vi "ex_setTdmProperty_I32.vi"(4 "Strings":string[](array[string]), 5 "Values":i32[](array[numeric]), 6 "Value":i32, 7 "Name":string) -> (3 "output cluster":T1)   [LabVIEW 2017]
uses:
  <vilib>/express/express shared/ExFile.llb/ex_TdmProperty.ctl
  <vilib>/express/express shared/ex_EditUserDefinedProperties/usiDataType.ctl
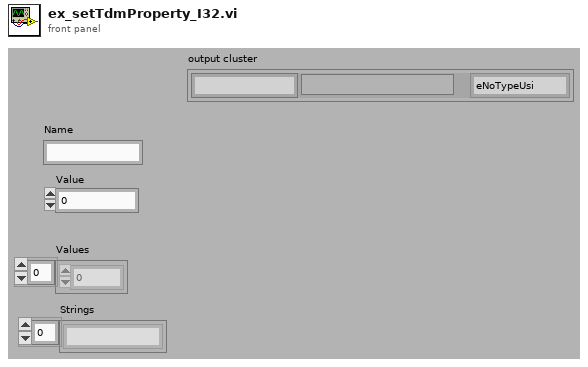
[diagram p1: front panel]
types:
  T1 = typedef "ex_TdmProperty.ctl" = cluster{"Name":string, "Type":T2, "Value":variant}
  T2 = typedef "usiDataType.ctl" = enum16{"eNoTypeUsi", "eInt8Usi", "eInt16Usi", "eInt32Usi", "eInt64Usi", "eUInt8Usi", "eUInt16Usi", "eUInt32Usi", "eUInt64Usi", "eFloat32Usi", "eFloat64Usi", "- 0", "- 1", "- 2", "- 3", "- 4", "- 5", "- 6", "- 7", "- 8", "- 9", "eString8Usi", "eString16Usi", "eStringUsi", "eEnumUsi", "- 10", "- 11", "- 12", "- 13", "- 14", "eTimeUsi", "- 15", "- 16", "- 17", "- 18", "- 19", "- 20", "- 21", "- 22", "- 23", "eInstanceUsi", "eStoreUsi"}
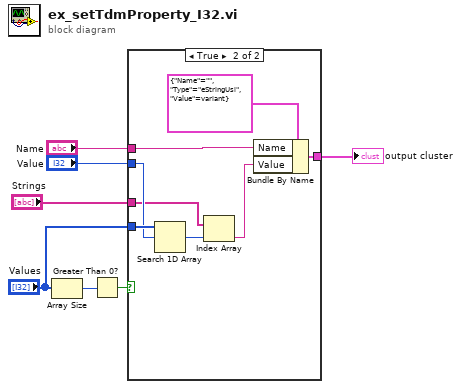
[diagram p0: block diagram]
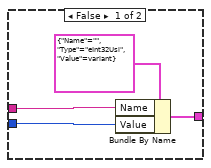
[diagram p2: hidden frame]
diagram:
  n1 = Array Size(array="Values") -> (size(s)=w4:i32)
  n2 = Greater Than 0?(x=w4) -> (x > 0?=w3:bool)
  n3 = case shown="True" w3 {
    tunnel: "Name" -> [w10 w18]
    tunnel: "Value" -> [w9 w15]
    tunnel: [w8 w17] -> w5
    tunnel: "Values" -> [_ w16]
    tunnel: "Strings" -> [_ w13]
    frame False {
      n4 = Bundle By Name(cluster=T1 {"Name"="", "Type"=enum."eInt32Usi", "Value"=variant} ("TDM Property"), "Name"=w10, "Value"=w9) -> (w8:T1)
    }
    frame True {
      n5 = Search 1D Array(1D array=w16, element=w15) -> (index of element=w14:i32)  [unwired: 1 in]
      n6 = Index Array(array=w13, index=w14) -> (element=w12:string)
      n7 = Bundle By Name(cluster=T1 {"Name"="", "Type"=enum."eStringUsi", "Value"=variant} ("TDM Property"), "Name"=w18, "Value"=w12) -> (w17:T1)
    }
  }
  "output cluster" <- w5
